vi "Get Multiple Attributes.vi"(0 "Attributes IN":variant, 7 "Attribute List":T1[](array[typedef])) -> (13 "Values":string[](array[string]), 14 "Attributes OUT":variant)   [LabVIEW 2020, in "GSwFormDSP.lvclass"]
uses:
  GSwFormDSP.lvclass
  functions/Attribute List.ctl
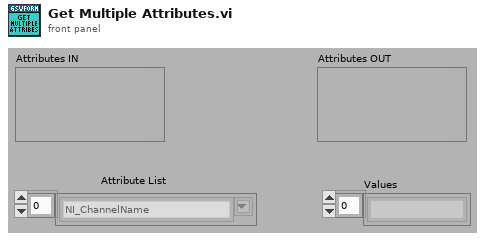
[diagram p1: front panel]
types:
  T1 = typedef "GSwFormDSP.lvclass/Attribute List.ctl" = string
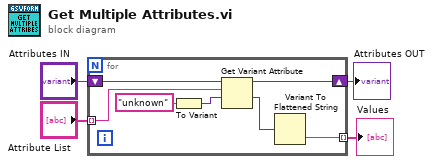
[diagram p0: block diagram]
diagram:
  n1 = for {
    shift-right: [w10] -> w3
    shift-left: "Attributes IN" -> [w11]
    tunnel: "Attribute List" -> [w9] mode=indexing
    tunnel: [w5] -> w1 mode=indexing
    n2 = To Variant(anything="unknown") -> (Variant=w7:variant)
    n3 = Get Variant Attribute(Variant=w11, name=w9, default value (empty Variant)=w7) -> (duplicate Variant=w10:variant, value=w6:variant)  [unwired: 1 in, 2 out]
    n4 = Variant To Flattened String(Variant=w6) -> (data string=w5:string)  [unwired: 1 out]
  }
  "Attributes OUT" <- w3
  "Values" <- w1
